vi "Get Network Adapter Settings.vi"(8 "error in":errorcluster, 11 "Refnum in":refnum<k21>) -> (0 "error out":errorcluster, 1 "Secondary Network Adapters":T1[](array[typedef]) {"IP Address Request Mode" items=["Static"=1, "DHCP/Link Local"=2, "Link-Local Only"=4, "DHCP Only"=8]; "Adapter Type" items=["Ethernet"=1, "WLAN"=2]; "Adapter Mode" items=["Disabled"=1, "TCP/IP Ethernet"=2, "Deterministic"=4, "EtherCAT"=8, "TCP/IP WLAN Connect"=32, "TCP/IP WLAN Create"=64]}, 2 "Primary Network Adapter":T1 {"IP Address Request Mode" items=["Static"=1, "DHCP/Link Local"=2, "Link-Local Only"=4, "DHCP Only"=8]; "Adapter Type" items=["Ethernet"=1, "WLAN"=2]; "Adapter Mode" items=["Disabled"=1, "TCP/IP Ethernet"=2, "Deterministic"=4, "EtherCAT"=8, "TCP/IP WLAN Connect"=32, "TCP/IP WLAN Create"=64]}, 3 "Refnum out":refnum<k21>)   [LabVIEW 2016, in "SMI.lvlib" / "Controller.lvclass"]
uses:
  Controller.lvclass
  Controls/NetworkAdapterSettings.ctl
  <vilib>/nisyscfg/Close (Hardware).vi
  <vilib>/nisyscfg/Find Hardware.vi
  <vilib>/nisyscfg/nisyscfg.lvlib
  <resource>/objmgr/niflexriosae.rc
  <resource>/objmgr/nicriosae.rc
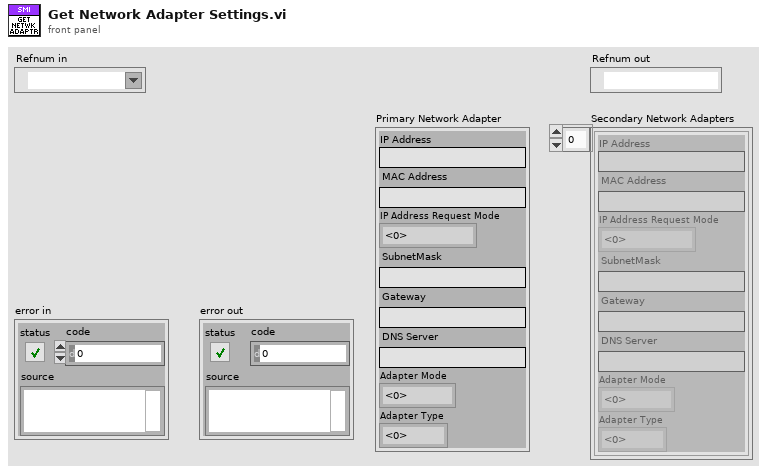
[diagram p1: front panel]
types:
  T1 = typedef "SMI.lvlib/Controller.lvclass/NetworkAdapterSettings.ctl" = cluster{"IP Address":string, "MAC Address":string, "IP Address Request Mode":u32, "SubnetMask":string, "Gateway":string, "DNS Server":string, "Adapter Mode":u32, "Adapter Type":u32}
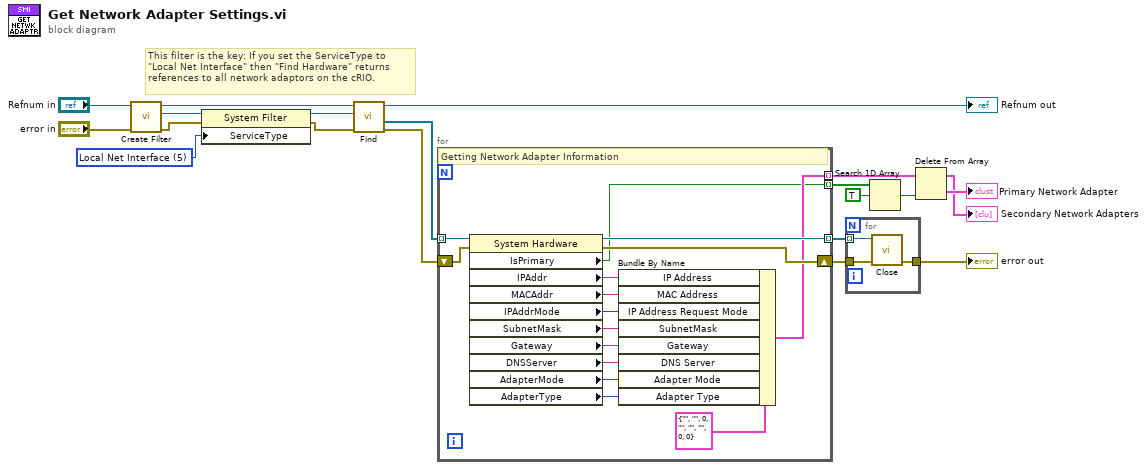
[diagram p0: block diagram]
diagram:
  w13 = u32 5 items=["NI Network Resource", "NI Real-Time", "NI System Configuration", "NI Web Interface", "Local System", "Local Net Interface", "Local Time Keeper", "Local Time Reference", "LXI Instrument"] ("Service Type")
  # "This filter is the key: If you set the ServiceType to\n\"Local Net Interface\" then \"Find Hardware\" returns\nreferences to all network adaptors on the cRIO."
  n1 = call <vilib>:"Create Filter.vi"("error in (no error)"="error in", "Session in"="Refnum in") -> ("error out"=w16:errorcluster, "Filter out"=w12:refnum<k20>, "Session out"=w11:refnum<k21>)  [unwired: 7 in]
  n2 = property class="System Filter"(reference=w12, error in=w16, "ServiceType"=w13) -> (reference out=w14:refnum<k20>, error out=w15:errorcluster)
  n3 = call-poly <vilib>:"Find.vi"("error in (no error)"=w15, "Filter in"=w14, "Session in"=w11) -> ("error out"=w17:errorcluster, "Resources out"=w7:refnum<k20>[], "Session out"=→"Refnum out":refnum<k21>)  [unwired: 5 in, 1 out]
  n4 = for {
    tunnel: w7 -> [w34] mode=indexing
    shift-right: [w23] -> w20
    shift-left: w17 -> [w35]
    tunnel: [w29] -> w10 mode=indexing
    tunnel: [w22] -> w6 mode=indexing
    tunnel: [w21] -> w5 mode=indexing
    # "Getting Network Adapter Information"
    n5 = property class="System Hardware"(reference=w34, error in=w35) -> (reference out=w29:refnum<k20>, error out=w23:errorcluster, "IsPrimary"=w21:bool, "IPAddr"=w24:string, "MACAddr"=w30:string, "IPAddrMode"=w27:u32, "SubnetMask"=w31:string, "Gateway"=w32:string, "DNSServer"=w33:string, "AdapterMode"=w26:u32, "AdapterType"=w25:u32)
    n6 = Bundle By Name(cluster=T1 {"IP Address"="", "MAC Address"="", "IP Address Request Mode"=0, "SubnetMask"="", "Gateway"="", "DNS Server"="", "Adapter Mode"=0, "Adapter Type"=0} ("Network Adapter Settings"), "IP Address"=w24, "MAC Address"=w30, "IP Address Request Mode"=w27, "SubnetMask"=w31, "Gateway"=w32, "DNS Server"=w33, "Adapter Mode"=w26, "Adapter Type"=w25) -> (w22:T1)
  }
  n7 = for {
    tunnel: [w38] -> w19
    tunnel: w20 -> [w37]
    tunnel: w10 -> [w36] mode=indexing
    n8 = call-poly <vilib>:"Close.vi"("error in (no error)"=w37, "Resource in"=w36) -> ("error out"=w38:errorcluster)  [unwired: 9 in]
  }
  "error out" <- w19
  n9 = Search 1D Array(1D array=w5, element=TRUE) -> (index of element=w3:i32)  [unwired: 1 in]
  n10 = Delete From Array(array=w6, index=w3) -> (deleted portion=→"Primary Network Adapter":T1, array with subset deleted=→"Secondary Network Adapters":T1[])  [unwired: 1 in]
